vi "Login_dialog.vi"() -> (0 "VISA resource name":refnum<visa-resource-name>="GPIB1::24::INSTR", 1 "Manual mode out":bool, 2 "Experiment title out":string, 3 "User name out":string)   [LabVIEW 2016]
panel:
  in  "Multiplexor":u16(ring) items=["QuickMUX", "None (manual mode)"]
  in  "Keithley model":u16(ring) items=["Keithley 2400", "Keithley 2450"]
  in  "Login":bool
  in  "Experiment title":string
  in  "User name":string
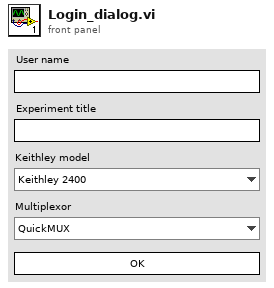
[diagram p1: front panel]
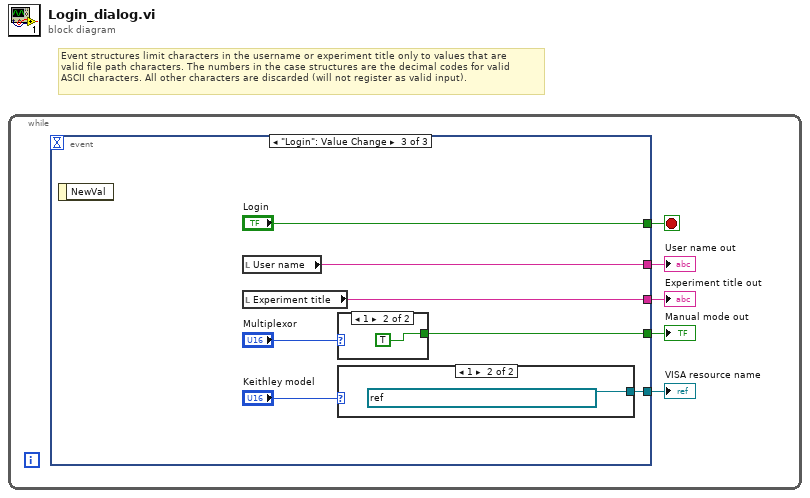
[diagram p0: block diagram]
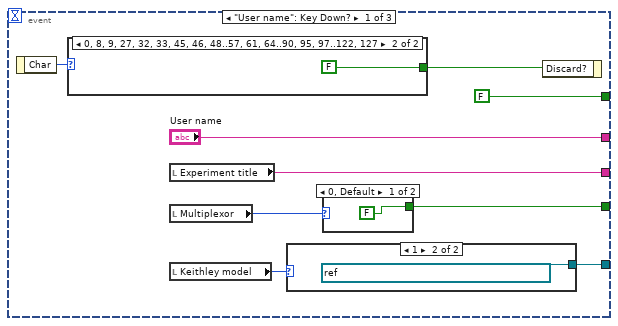
[diagram p2: hidden frame]
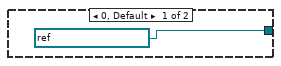
[diagram p3: hidden frame]
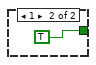
[diagram p4: hidden frame]
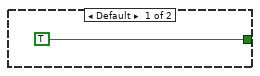
[diagram p5: hidden frame]
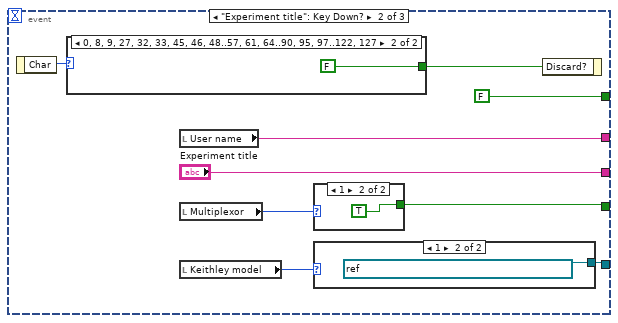
[diagram p6: hidden frame]
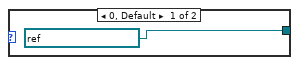
[diagram p7: hidden frame]
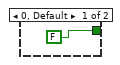
[diagram p8: hidden frame]
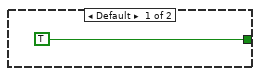
[diagram p9: hidden frame]
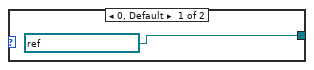
[diagram p10: hidden frame]
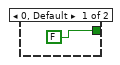
[diagram p11: hidden frame]
diagram:
  # "Event structures limit characters in the username or experiment title only to values that are\nvalid file path characters. The numbers in the case structures are the decimal codes for valid\nASCII characters. All other characters are discarded (will not register as valid input)."
  n1 = while {
    stop <- w5 stop-if-true
    n2 = event shown="[2] \"Login\": Value Change" {
      selector: _ -> [_ _ _]
      dyn-events: _ -> [_ _ _]
      timeout: _ -> [_ _ _]
      tunnel: [FALSE ("NewVal") FALSE ("NewVal") "Login"] -> w5
      tunnel: ["User name" w26 w41] -> w4
      tunnel: [w10 "Experiment title" w40] -> w3
      tunnel: [w9 w24 w38] -> w2
      tunnel: [w8 w23 w36] -> w1
      event "User name": Key Down? {
        n3 = event-data() -> ("Char"=w14:i16)  [unwired: 1 in]
        n4 = case shown="0, 8, 9, 27, 32, 33, 45, 46, 48..57, 61, 64..90, 95, 97..122, 127" w14 {
          tunnel: [TRUE FALSE] -> w13
          frame Default {
          }
          frame 0, 8, 9, 27, 32, 33, 45, 46, 48..57, 61, 64..90, 95, 97..122, 127 {
          }
        }
        n5 = local read "Experiment title"() -> (w10:string)
        n6 = local read "Multiplexor"() -> (w6:u16)
        n7 = local read "Keithley model"() -> (w7:u16)
        n8 = case shown="1" w7 {
          tunnel: [refnum<visa-resource-name> "GPIB1::24::INSTR" ("VISA resource name") refnum<visa-resource-name> "USB0::0x05E6::0x2450::04049675::INSTR" ("VISA resource name")] -> w8
          frame 0, Default {
          }
          frame 1 {
          }
        }
        n9 = case shown="0, Default" w6 {
          tunnel: [FALSE ("Manual mode out 2") TRUE ("Manual mode out 2")] -> w9
          frame 0, Default {
          }
          frame 1 {
          }
        }
        n10 = event-data("Discard?"=w13) -> ()  [unwired: 1 in, 1 out]
      }
      event "Experiment title": Key Down? {
        n11 = event-data() -> ("Char"=w29:i16)  [unwired: 1 in]
        n12 = case shown="0, 8, 9, 27, 32, 33, 45, 46, 48..57, 61, 64..90, 95, 97..122, 127" w29 {
          tunnel: [TRUE FALSE] -> w28
          frame Default {
          }
          frame 0, 8, 9, 27, 32, 33, 45, 46, 48..57, 61, 64..90, 95, 97..122, 127 {
          }
        }
        n13 = local read "User name"() -> (w26:string)
        n14 = local read "Multiplexor"() -> (w22:u16)
        n15 = local read "Keithley model"() -> (w21:u16)
        n16 = case shown="1" w22 {
          tunnel: [FALSE ("Manual mode out 2") TRUE ("Manual mode out 2")] -> w24
          frame 0, Default {
          }
          frame 1 {
          }
        }
        n17 = case shown="1" w21 {
          tunnel: [refnum<visa-resource-name> "GPIB1::24::INSTR" ("VISA resource name") refnum<visa-resource-name> "USB0::0x05E6::0x2450::04049675::INSTR" ("VISA resource name")] -> w23
          frame 0, Default {
          }
          frame 1 {
          }
        }
        n18 = event-data("Discard?"=w28) -> ()  [unwired: 1 in, 1 out]
      }
      event "Login": Value Change {
        n19 = event-data() -> ()  [unwired: 1 in, 1 out]
        n20 = local read "User name"() -> (w41:string)
        n21 = local read "Experiment title"() -> (w40:string)
        n22 = case shown="1" "Multiplexor" {
          tunnel: [FALSE ("Manual mode out 2") TRUE ("Manual mode out 2")] -> w38
          frame 0, Default {
          }
          frame 1 {
          }
        }
        n23 = case shown="1" "Keithley model" {
          tunnel: [refnum<visa-resource-name> "GPIB1::24::INSTR" ("VISA resource name") refnum<visa-resource-name> "USB0::0x05E6::0x2450::04049675::INSTR" ("VISA resource name")] -> w36
          frame 0, Default {
          }
          frame 1 {
          }
        }
      }
    }
    "User name out" <- w4
    "Experiment title out" <- w3
    "Manual mode out" <- w2
    "VISA resource name" <- w1
  }
